vi "Length_1Eje.vi"(1 "Dist_Eje":i32) -> (0 "Dist_EjeSTR":string)   [LabVIEW 2021]
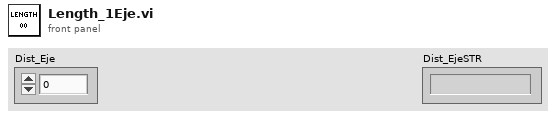
[diagram p1: front panel]
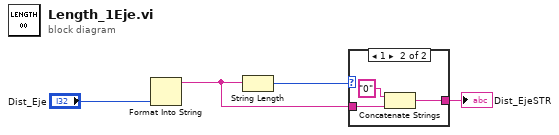
[diagram p0: block diagram]
diagram:
  n1 = Format Into String("Dist_Eje") -> (resulting string=w2:string)  [unwired: 3 in, 1 out]
  n2 = String Length(string=w2) -> (length=w3:i32)
  n3 = case shown="1" w3 {
    tunnel: w2 -> [w5 w8]
    tunnel: [w5 w6] -> w1
    frame 2, Default {
    }
    frame 1 {
      n4 = Concatenate Strings("0" ("string"), w8) -> (w6:string)
    }
  }
  "Dist_EjeSTR" <- w1
